vi "Cross Product.vi"(10 "Vector B":T1, 11 "Vector A":T1) -> (3 "Cross Product":T1)   [LabVIEW 2020, in "3D (FPGA).lvlib"]
uses:
  3D (FPGA).lvlib
  Vector 3D.ctl
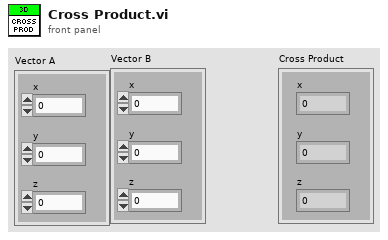
[diagram p1: front panel]
types:
  T1 = typedef "3D (FPGA).lvlib/Vector 3D.ctl" = cluster{"x":sgl, "y":sgl, "z":sgl}
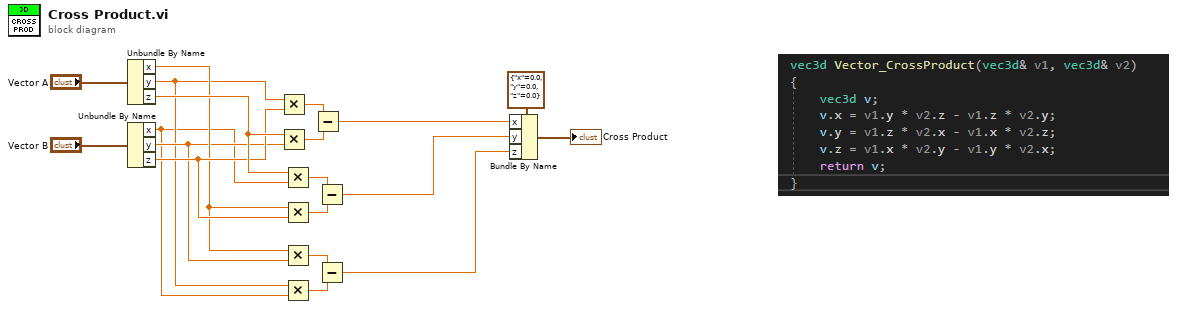
[diagram p0: block diagram]
diagram:
  n1 = Unbundle By Name("Vector A") -> ("x"=w4:sgl, "y"=w2:sgl, "z"=w6:sgl)
  n2 = Unbundle By Name("Vector B") -> ("x"=w1:sgl, "y"=w3:sgl, "z"=w5:sgl)
  n3 = Multiply(x=w2, y=w5) -> (x*y=w17:sgl)
  n4 = Multiply(x=w6, y=w3) -> (x*y=w13:sgl)
  n5 = Multiply(x=w6, y=w1) -> (x*y=w11:sgl)
  n6 = Multiply(x=w4, y=w5) -> (x*y=w12:sgl)
  n7 = Multiply(x=w4, y=w3) -> (x*y=w10:sgl)
  n8 = Multiply(x=w2, y=w1) -> (x*y=w9:sgl)
  n9 = Subtract(x=w17, y=w13) -> (x-y=w14:sgl)
  n10 = Subtract(x=w11, y=w12) -> (x-y=w8:sgl)
  n11 = Subtract(x=w10, y=w9) -> (x-y=w7:sgl)
  n12 = Bundle By Name(cluster=T1 {"x"=0.0, "y"=0.0, "z"=0.0} ("Cross Product"), "x"=w14, "y"=w8, "z"=w7) -> (→"Cross Product":T1)
